vi "PH_PILS.vis MainAmpEnablingKnob.vi"(0 "i ref in":refnum<vi>, 5 "error IO":errorcluster) -> (14 "i ref out":refnum<vi>, 19 "error out":errorcluster)   [LabVIEW 2014, in "PH_PILS.lvlib"]
uses:
  PH_PILS.lvlib
  PH_PILS.Submode.ctl
  PH_SystemInformation/PH_SystemInformation.lvlib
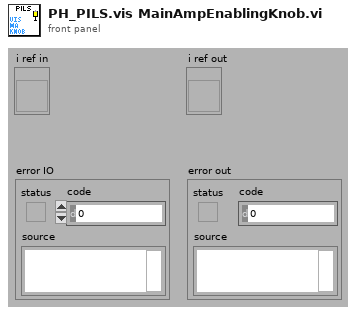
[diagram p1: front panel]
types:
  T1 = typedef "PH_PILS.lvlib/PH_PILS.Submode.ctl" = enum16{"unknown", "HV-Normal", "HV-Test"}
  T2 = typedef "PH_PILS.lvlib/PH_PILS.i attribute.ctl" = cluster{"Boolean":cluster{"GUI Ref":refnum<vi>, "Status":i32}[], "GUI Refs Exp. Shutters":cluster{"1":refnum<vi>, "2":refnum<vi>, "3":refnum<vi>, "4":refnum<vi>}, "Tristate2Run GUI Refs":refnum<vi>[], "EO-Likes":cluster{"GUI Ref":refnum<vi>, "Status":i32}[], "Operation Mode":cluster{"Operation Mode":T3, "GUI":cluster{"Ref State":refnum<vi>, "Ref":refnum<vi>}, "Servicemode":cluster{"Tagname":string, "Status":i32}, "Labormode":cluster{"Tagname":string, "Status":i32}, "Searchmode":cluster{"Tagname":string, "Status":i32}, "Shotmode":cluster{"Tagname":string, "Status":i32}}, "Submode":cluster{"Submode":T1, "GUI":cluster{"Ref State":refnum<vi>, "Ref":refnum<vi>}, "Submode":cluster{"Tagname":string, "Status":i32}}, "Experiment":cluster{"Experiment":enum16{"unknown", "intern", "4 (Z6)", "3", "2", "1"}, "GUI":cluster{"Ref State":refnum<vi>, "Ref":refnum<vi>}, "intern":cluster{"Tagname":string, "Status":i32}, "Exp 4":cluster{"Tagname":string, "Status":i32}, "Exp 3":cluster{"Tagname":string, "Status":i32}, "Exp 2":cluster{"Tagname":string, "Status":i32}, "Exp 1":cluster{"Tagname":string, "Status":i32}}, "TristateNormal":cluster{"GUI Ref":refnum<vi>, "Status":i32}[], "Door Tags":cluster{"GUI Ref":refnum<vi>, "Status":i32}[], "GUIlessTags":cluster{"Name":string, "Status":i32}[], "Beamline GUI Refs":refnum<vi>[], "Special Boolean":cluster{"GUI Ref":refnum<vi>, "Status":i32}[], "Laserpower":cluster{"GUI Ref":refnum<vi>, "Status":i32}[], "Shutter":cluster{"GUI Ref":refnum<vi>, "Status":i32}[], "Tristate EO Like":cluster{"GUI Ref":refnum<vi>, "Status":i32}[], "PP":cluster{"GUI Ref":refnum<vi>, "Status":i32, "Head Ref":refnum<vi>, "Slider Ref":refnum<vi>}[], "Switch Knobs":cluster{"GUI Ref":refnum<vi>, "Status":i32}[], "Latch Knob GUI Refs":refnum<vi>[], "FailureCounter":i32, "Enabled Status":cluster{"Laser":i32, "PreAmp":i32, "MainAmp":i32}, "Mercury":refnum<vi>, "Instance Rods":string, "Logfile":path, "Beckhoff-Instance Internal":string, "Beckhoff-Instance External":string, "Enabling Rights":cluster{"Name":string, "Password":string, "PA?":bool, "MA?":bool, "Exp?":bool}[]}
  T3 = typedef "PH_PILS.lvlib/PH_PILS.Operation Mode.ctl" = enum16{"unknown", "Service", "Labor", "Search", "Shot"}
  T4 = enum16{"unknown", "intern", "4 (Z6)", "3", "2", "1"}
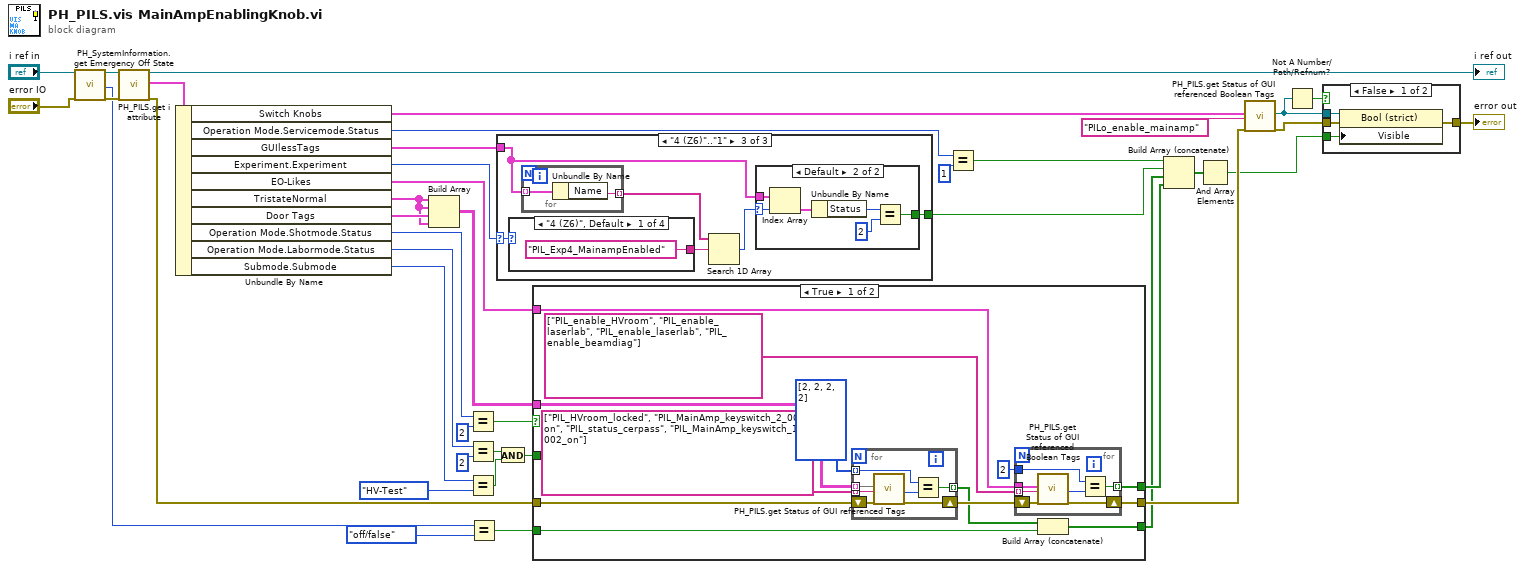
[diagram p0: block diagram]
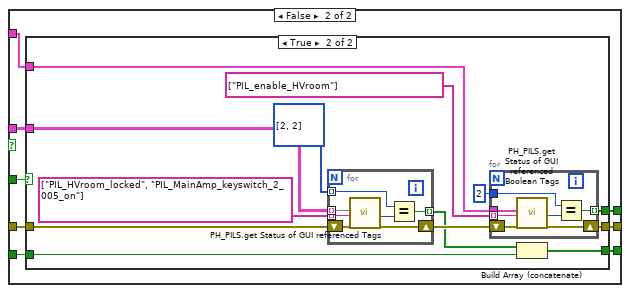
[diagram p2: hidden frame]
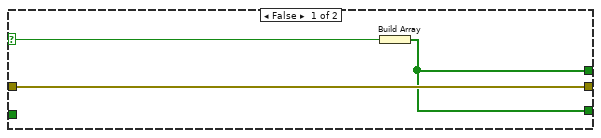
[diagram p3: hidden frame]
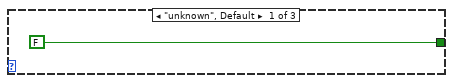
[diagram p4: hidden frame]
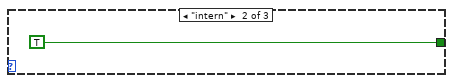
[diagram p5: hidden frame]
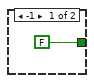
[diagram p6: hidden frame]
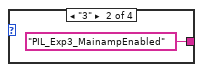
[diagram p7: hidden frame]
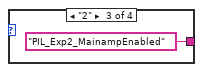
[diagram p8: hidden frame]
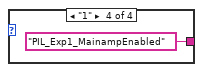
[diagram p9: hidden frame]
diagram:
  n1 = call "PH_SystemInformation.get Emergency Off State.vi"("i ref in"="i ref in", "error in (no error)"="error IO") -> ("i ref out"=w6:refnum<vi>, "Emergency Off State"=w3:enum16{"no info", "off/false", "Alarm"}, "error out"=w4:errorcluster)  [unwired: 15 in]
  n2 = call "PH_PILS.get i attribute.vi"("i ref in"=w6, "error in (no error)"=w4) -> ("i ref out"=→"i ref out":refnum<vi>, "i attribute"=w40:T2, "error out"=w28:errorcluster)  [unwired: 15 in]
  n3 = Unbundle By Name(w40) -> ("Switch Knobs"=w39:cluster{"GUI Ref":refnum<vi>, "Status":i32}[], "Operation Mode.Servicemode.Status"=w32:i32, "GUIlessTags"=w23:cluster{"Name":string, "Status":i32}[], "Experiment.Experiment"=w19:T4, "EO-Likes"=w18:cluster{"GUI Ref":refnum<vi>, "Status":i32}[], "TristateNormal"=w24:cluster{"GUI Ref":refnum<vi>, "Status":i32}[], "Door Tags"=w33:cluster{"GUI Ref":refnum<vi>, "Status":i32}[], "Operation Mode.Shotmode.Status"=w16:i32, "Operation Mode.Labormode.Status"=w13:i32, "Submode.Submode"=w12:T1)
  n4 = Build Array(w24, w24, w33, w24) -> (w17:cluster{"GUI Ref":refnum<vi>, "Status":i32}[][])
  n5 = Equal?(x=w16, y=2) -> (x = y?=w15:bool)
  n6 = Equal?(x=w13, y=2) -> (x = y?=w10:bool)
  n7 = Equal?(x=w12, y=PH_PILS.Submode."HV-Test" ("Submode.Submode")) -> (x = y?=w9:bool)
  n8 = Equal?(x=w3, y=enum16{"no info", "off/false", "Alarm"}."off/false" ("Emergency Off State")) -> (x = y?=w1:bool)
  n9 = case shown="\"4 (Z6)\"..\"1\"" w19 {
    selector: w19 -> [_ _ w48]
    tunnel: w23 -> [_ _ w45]
    tunnel: [FALSE TRUE w46] -> w20
    frame "unknown", Default {
    }
    frame "intern" {
    }
    frame "4 (Z6)".."1" {
      n10 = case shown="\"4 (Z6)\", Default" w48 {
        tunnel: ["PIL_Exp4_MainampEnabled" "PIL_Exp3_MainampEnabled" "PIL_Exp2_MainampEnabled" "PIL_Exp1_MainampEnabled"] -> w47
        frame "4 (Z6)", Default {
        }
        frame "3" {
        }
        frame "2" {
        }
        frame "1" {
        }
      }
      n11 = for {
        tunnel: w45 -> [w62] mode=indexing
        tunnel: [w61] -> w49 mode=indexing
        n12 = Unbundle By Name(w62) -> ("Name"=w61:string)
      }
      n13 = Search 1D Array(1D array=w49, element=w47) -> (index of element=w44:i32)  [unwired: 1 in]
      n14 = case shown="Default" w44 {
        selector: w44 -> [_ w51]
        tunnel: [FALSE w53] -> w46
        tunnel: w45 -> [_ w52]
        frame -1 {
        }
        frame Default {
          n15 = Index Array(array=w52, index=w51) -> (element=w56:cluster{"Name":string, "Status":i32})
          n16 = Unbundle By Name(w56) -> ("Status"=w55:i32)
          n17 = Equal?(x=w55, y=2) -> (x = y?=w53:bool)
        }
      }
    }
  }
  n18 = And(x=w10, y=w9) -> (x .and. y?=w8:bool)
  n19 = case shown="True" w15 {
    tunnel: [w72 w97] -> w29
    tunnel: w28 -> [w71 w96]
    tunnel: [w68 w95] -> w25
    tunnel: [w65 w94] -> w22
    tunnel: w18 -> [w67 w93]
    tunnel: w17 -> [w66 w92]
    tunnel: w8 -> [_ w91]
    tunnel: w1 -> [w63 w90]
    frame True {
      n20 = for {
        tunnel: string[] ["PIL_HVroom_locked", "PIL_MainAmp_keyswitch_2_005_on", "PIL_status_cerpass", "PIL_MainAmp_keyswitch_1_002_on"] -> [w89] mode=indexing
        shift-right: [w88] -> w73
        shift-left: w71 -> [w87]
        tunnel: w66 -> [w86] mode=indexing
        tunnel: i32[] [2, 2, 2, 2] -> [w84] mode=indexing
        tunnel: [w85] -> w64 mode=indexing
        n21 = call "PH_PILS.get Status of GUI referenced Tags.vi"("Tags"=w86, "Tagname"=w89, "error in"=w87) -> ("Status"=w83:i32, "error out"=w88:errorcluster)  [unwired: 13 in, 2 out]
        n22 = Equal?(x=w84, y=w83) -> (x = y?=w85:bool)
      }
      n23 = for {
        tunnel: w67 -> [w80]
        tunnel: string[] ["PIL_enable_HVroom", "PIL_enable_laserlab", "PIL_enable_laserlab", "PIL_enable_beamdiag"] -> [w79] mode=indexing
        shift-right: [w81] -> w72
        shift-left: w73 -> [w82]
        tunnel: [w77] -> w68 mode=indexing
        tunnel: 2 ("x") -> [w76]
        n24 = call "PH_PILS.get Status of GUI referenced Boolean Tags.vi"("Tags"=w80, "Tagname"=w79, "error in"=w82) -> ("Status"=w78:i32, "error out"=w81:errorcluster)  [unwired: 13 in, 2 out]
        n25 = Equal?(x=w76, y=w78) -> (x = y?=w77:bool)
      }
      n26 = Build Array (concatenate)(w64, w63) -> (w65:bool[])
    }
    frame False {
      n27 = case shown="True" w91 {
        selector: w91 -> [w99 _]
        tunnel: [w100 w110] -> w97
        tunnel: w96 -> [w100 w109]
        tunnel: [w98 w106] -> w95
        tunnel: [w98 w102] -> w94
        tunnel: w93 -> [_ w105]
        tunnel: w92 -> [_ w104]
        tunnel: w90 -> [_ w103]
        frame False {
          n28 = Build Array(w99) -> (w98:bool[])
        }
        frame True {
          n29 = for {
            tunnel: string[] ["PIL_HVroom_locked", "PIL_MainAmp_keyswitch_2_005_on"] -> [w127] mode=indexing
            shift-right: [w126] -> w111
            shift-left: w109 -> [w125]
            tunnel: w104 -> [w124] mode=indexing
            tunnel: i32[] [2, 2] -> [w122] mode=indexing
            tunnel: [w123] -> w101 mode=indexing
            n30 = call "PH_PILS.get Status of GUI referenced Tags.vi"("Tags"=w124, "Tagname"=w127, "error in"=w125) -> ("Status"=w121:i32, "error out"=w126:errorcluster)  [unwired: 13 in, 2 out]
            n31 = Equal?(x=w122, y=w121) -> (x = y?=w123:bool)
          }
          n32 = for {
            tunnel: w105 -> [w118]
            tunnel: string[] ["PIL_enable_HVroom"] -> [w117] mode=indexing
            shift-right: [w119] -> w110
            shift-left: w111 -> [w120]
            tunnel: [w115] -> w106 mode=indexing
            tunnel: 2 ("x") -> [w114]
            n33 = call "PH_PILS.get Status of GUI referenced Boolean Tags.vi"("Tags"=w118, "Tagname"=w117, "error in"=w120) -> ("Status"=w116:i32, "error out"=w119:errorcluster)  [unwired: 13 in, 2 out]
            n34 = Equal?(x=w114, y=w116) -> (x = y?=w115:bool)
          }
          n35 = Build Array (concatenate)(w101, w103) -> (w102:bool[])
        }
      }
    }
  }
  n36 = Equal?(x=w32, y=1) -> (x = y?=w21:bool)
  n37 = Build Array (concatenate)(w21, w20, w22, w25) -> (w27:bool[])
  n38 = And Array Elements(Boolean array=w27) -> (logical AND=w26:bool)
  n39 = call "PH_PILS.get Status of GUI referenced Boolean Tags.vi"("Tags"=w39, "Tagname"="PILo_enable_mainamp", "error in"=w29) -> ("GUI Ref"=w36:refnum<vi>, "error out"=w38:errorcluster)  [unwired: 13 in, 2 out]
  n40 = Not A Number/Path/Refnum?(number/path/refnum=w36) -> (NaN/Path/Refnum?=w37:bool)
  n41 = case shown="False" w37 {
    tunnel: w38 -> [w131 w132]
    tunnel: w36 -> [w130 _]
    tunnel: [w129 w132] -> w35
    tunnel: w26 -> [w128 _]
    frame False {
      n42 = property class="Bool (strict)"(reference=w130, error in=w131, "Visible"=w128) -> (error out=w129:errorcluster)  [unwired: 1 out]
    }
    frame True {
    }
  }
  "error out" <- w35
